vi "Read ext.vi"(8 "error in":errorcluster, 11 "PAS Cell Data in":refnum<class "PAS Cell Data.lvclass">) -> (0 "error out":errorcluster, 2 "ext":dbl, 3 "PAS Cell Data out":refnum<class "PAS Cell Data.lvclass">)   [LabVIEW 2015, in "PAS Library.lvlib" / "PAS Cell Data.lvclass"]
uses:
  PAS Cell Data.lvclass
  PAS Cell Data.lvclass/PAS Cell Data.ctl
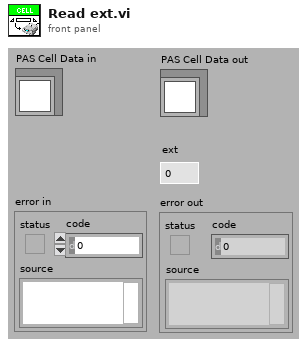
[diagram p1: front panel]
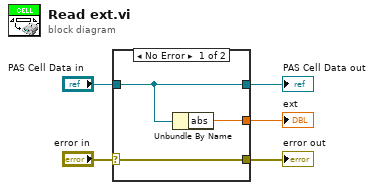
[diagram p0: block diagram]
diagram:
  n1 = case shown="No Error" "error in" {
    selector: "error in" -> [w8 w9]
    tunnel: [w8 w9] -> w4
    tunnel: [w7 w10] -> w2
    tunnel: "PAS Cell Data in" -> [w7 w10]
    tunnel: [w6 _] -> w1
    frame No Error {
      n2 = Unbundle By Name(w7) -> ("abs"=w6:dbl)
    }
    frame Error {
    }
  }
  "error out" <- w4
  "PAS Cell Data out" <- w2
  "ext" <- w1
